vi "Close.vi"(8 "error in (no error)":errorcluster caption="entrée d'erreur (pas d'erreur)", 11 "Class UART Nodon.lvclass En entrée":refnum<class "Class UART Nodon.lvclass">) -> (0 "error out":errorcluster caption="sortie d'erreur", 3 "Class UART Nodon.lvclass En sortie":refnum<class "Class UART Nodon.lvclass">)   [LabVIEW 2020, in "Library Instrument & Equipement.lvlib" / "Library UART.lvlib" / "Class UART Nodon.lvclass"]
uses:
  Class UART Nodon.lvclass
  Commun VI/TypeDef/Variable Printable.ctl
  UART (Default)/Class UART (Default).lvclass
  Commun VI/Library Commun.lvlib
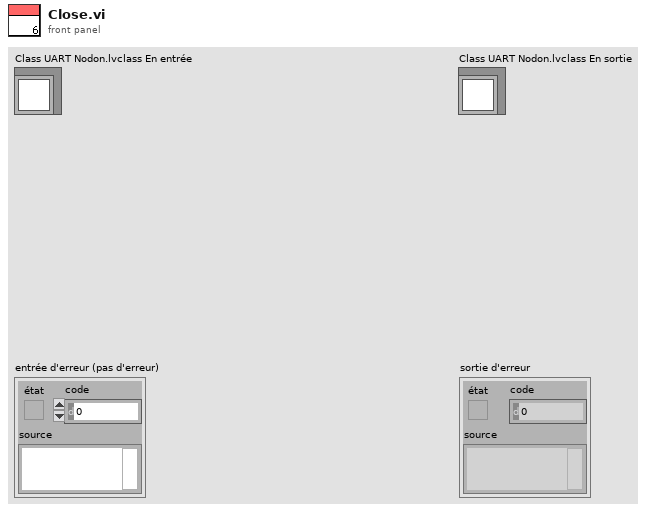
[diagram p1: front panel]
types:
  T1 = typedef "Variable Printable.ctl" = string
  T2 = enum16{"Get Variable", "Get All Variables", "Set Variable", "Delete Variable", "Delete All Variable"}
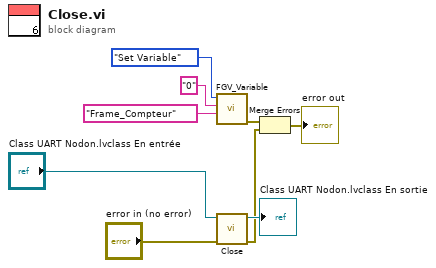
[diagram p0: block diagram]
diagram:
  n1 = call "FGV_Variable.vi"("Variable"=T1 "Frame_Compteur", "Data In"="0", "Function"=T2."Set Variable") -> ("error out"=w3:errorcluster)  [unwired: 6 in, 2 out]
  n2 = call-parent "Close.vi"("error in (no error)"="error in (no error)", "Class UART (Default) en entrée"="Class UART Nodon.lvclass En entrée") -> ("error out"=w1:errorcluster, "Class UART (Default) en sortie"=→"Class UART Nodon.lvclass En sortie":refnum<class "Class UART Nodon.lvclass">)  [unwired: 8 in]
  n3 = Merge Errors(w3, w1) -> (→"error out":errorcluster)
